vi "ROS_Topic_Close.vi"(0 "error in":errorcluster, 2 "topic":string, 3 "StopConsole":bool=TRUE) -> (1 "error out":errorcluster)   [LabVIEW 2010]
doc: "Closes a topic. If no topic is defined, it will close all tasks and close the console (unless specified otherwise)."
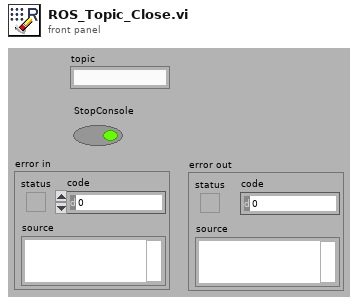
[diagram p1: front panel]
types:
  T1 = enum16{"Add Server", "Clear Server", "Clear All", "Get Info"}
  T2 = typedef "ServoInfo.ctl" = cluster{"vi name":string, "VI Refnum":refnum<vi>, "queue":refnum<queue>, "ROS":T3, "notifier":refnum<notifier>}
  T3 = typedef "_ROSControl.ctl" = cluster{"topic port":u16, "Node":string, "topic":string, "type":string, "node port":u32, "error ":errorcluster, "Direction":T4, "APIs":string[], "Update (ms)":u16, "write queue":u16}
  T4 = typedef "_ROSDirection.ctl" = enum16{"Node", "Publisher", "Subscriber", "Service Client"}
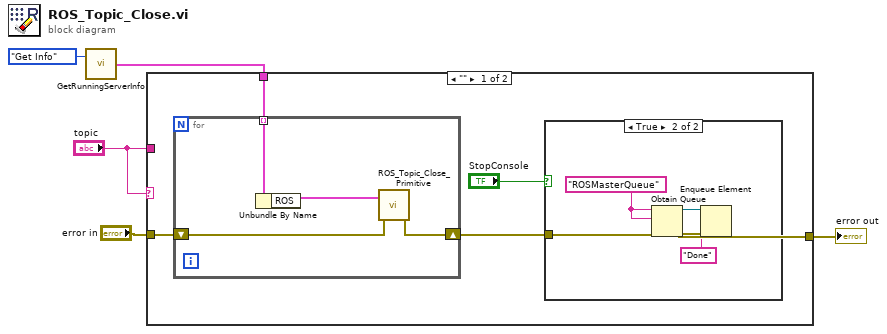
[diagram p0: block diagram]
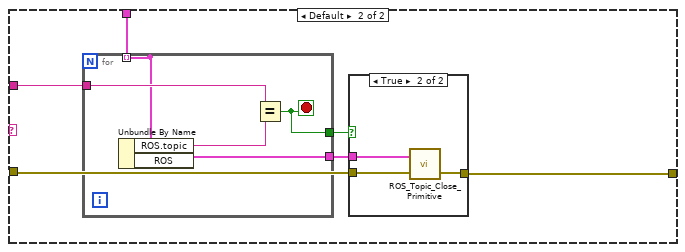
[diagram p3: hidden frame]
diagram:
  n1 = call "GetRunningServerInfo.vi"("Task"=T1."Get Info") -> ("servers"=w1:T2[])  [unwired: 1 in, 2 out]
  n2 = case shown="\"\"" "topic" {
    tunnel: "topic" -> [_ w23]
    tunnel: [w8 w22] -> w5
    tunnel: "error in" -> [w7 w21]
    tunnel: w1 -> [w6 w20]
    frame "" {
      n3 = for {
        shift-right: [w17] -> w8
        shift-left: w7 -> [w18]
        tunnel: w6 -> [w16] mode=indexing
        n4 = Unbundle By Name(w16) -> ("ROS"=w15:T3)
        n5 = call "ROS_Topic_Close_Primitive.vi"("error in"=w18, "ROS in"=w15) -> ("error out"=w17:errorcluster)  [unwired: 1 in]
      }
      n6 = case shown="True" "StopConsole" {
        tunnel: w8 -> [_ w11]
        frame False {
        }
        frame True {
          w13 = "ROSMasterQueue" ("name (unnamed)")
          n7 = Obtain Queue(name (unnamed)=w13, element data type=w13, error in (no error)=w11) -> (queue out=w14:refnum<queue>, error out=w10:errorcluster)  [unwired: 2 in, 1 out]
          n8 = Enqueue Element(queue=w14, element="Done", error in (no error)=w10) -> ()  [unwired: 1 in, 3 out]
        }
      }
    }
    frame Default {
      n9 = for {
        tunnel: w23 -> [w33]
        tunnel: [w32] -> w24
        tunnel: [w31] -> _ mode=indexing
        tunnel: w20 -> [w31] mode=indexing
        tunnel: [w30] -> w19
        stop <- w32 stop-if-true
        n10 = Unbundle By Name(w31) -> ("ROS.topic"=w29:string, "ROS"=w30:T3)
        n11 = Equal?(x=w33, y=w29) -> (x = y?=w32:bool)
      }
      n12 = case shown="True" w24 {
        tunnel: [w25 w28] -> w22
        tunnel: w21 -> [w25 w27]
        tunnel: w19 -> [_ w26]
        frame False {
        }
        frame True {
          n13 = call "ROS_Topic_Close_Primitive.vi"("error in"=w27, "ROS in"=w26) -> ("error out"=w28:errorcluster)  [unwired: 1 in]
        }
      }
    }
  }
  "error out" <- w5
